vi "ErrorLog.vi"(7 "ErrorLogMode":T1=enum."Add", 8 "error in (no error)":errorcluster caption="エラー入力（エラーなし）", 10 "ModuleName":string="Manager") -> (0 "error out":errorcluster caption="エラー出力", 3 "path":path)   [LabVIEW 2021]
doc: "ErrorLogを保存します。\nInitモードで初期化時にログファイルを作成します。\nログファイルはユーザードキュメントフォルダ内の”ModuleName”のフォルダにErrorLog20210227.txtなどの名称で作成します。（20210527は作成年月日）\nAddモード時にエラー入力にエラーが入力されると上記ファイルに保存します。\n保存する項目は、日付_時刻（年月日_時分秒）、エラーCode、エラーソースです。\nエラーログファイルは、書き込み時に毎回、開く、閉じるの操作を行います。\n大量のエラーが連続して発生すると書き込み処理が追いつかなくなる恐れが有ります。"
uses:
  ErrorLogMode.ctl
  <vilib>/Utility/sysdir.llb/System Directory Type.ctl
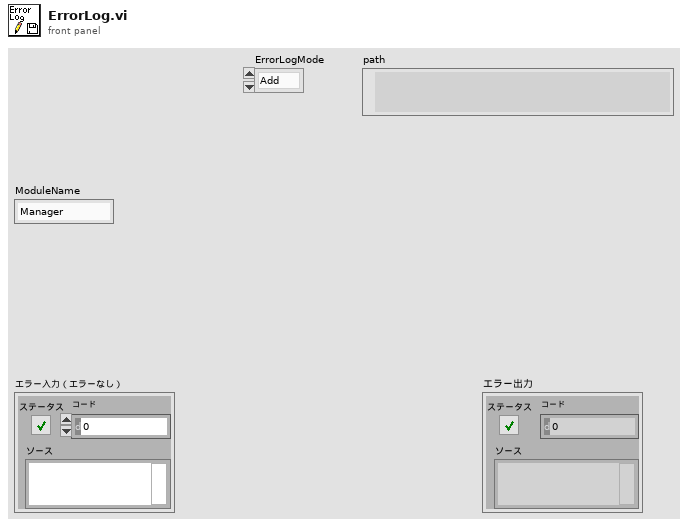
[diagram p1: front panel]
types:
  T1 = typedef "ErrorLogMode.ctl" = enum16{"Init", "Add"}
  T2 = enum16{"open", "replace", "create", "open or create", "replace or create", "replace or create with confirmation"}
  T3 = typedef "System Directory Type.ctl" = i32
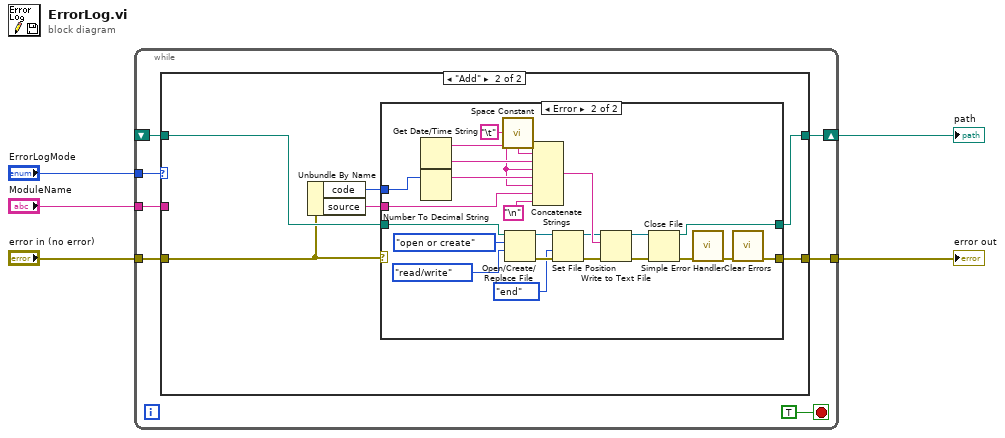
[diagram p0: block diagram]
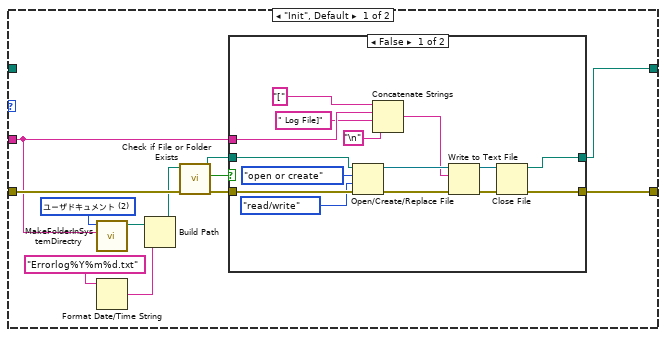
[diagram p2: hidden frame]
diagram:
  n1 = while {
    tunnel: "ErrorLogMode" -> [w11]
    tunnel: "error in (no error)" -> [w10]
    tunnel: [w9] -> w3
    shift-right: [w8] -> w1
    shift-left: _ -> [w7]
    tunnel: "ModuleName" -> [w6]
    stop <- TRUE stop-if-true
    n2 = case shown="\"Add\"" w11 {
      tunnel: w10 -> [w24 w42]
      tunnel: [w22 w47] -> w9
      tunnel: [w20 w46] -> w8
      tunnel: w7 -> [_ w43]
      tunnel: w6 -> [w13 _]
      frame "Init", Default {
        w15 = T3 2 items=["ユーザホーム"=0, "ユーザデスクトップ"=1, "ユーザドキュメント"=2, "ユーザアプリケーションデータ"=3, "ユーザ設定"=4, "ユーザ一時"=5, "パブリックドキュメント"=6, "パブリックアプリケーションデータ"=7, "パブリック環境設定"=8, "パブリックキャッシュ"=13, "システムコアライブラリ"=9, "システムインストールされたライブラリ"=10, "アプリケーションファイル"=11, "ブート容量ルート"=12] ("system directory type")
        n3 = call "MakeFolderInSystemDirectry.vi"("名前または相対パス"=w13, "system directory type"=w15) -> ("dup path"=w17:path)  [unwired: 8 in, 1 out]
        n4 = Format Date/Time String(time format string (%c)="Errorlog%Y%m%d.txt" ("名前または相対パス")) -> (date/time string=w18:string)  [unwired: 2 in]
        n5 = Build Path(base path=w17, name or relative path=w18) -> (appended path=w14:path)
        n6 = call <vilib>:"Check if File or Folder Exists.vi"("error in (no error)"=w24, "path"=w14) -> ("error out"=w21:errorcluster, "file or folder exists?"=w23:bool, "dup path"=w19:path)  [unwired: 7 in]
        n7 = case shown="False" w23 {
          tunnel: [w35 w41] -> w22
          tunnel: w21 -> [w39 w41]
          tunnel: [w32 w40] -> w20
          tunnel: w19 -> [w33 w40]
          tunnel: w13 -> [w27 _]
          frame False {
            n8 = Open/Create/Replace File(file path (use dialog)=w33, error in=w39, operation (0:open)=T2."open or create" ("操作（0:open）"), access (0:read/write)=enum16{"read/write", "read-only", "write-only"}."read/write" ("アクセス（0:read/write）")) -> (refnum out=w34:refnum<file>, error out=w38:errorcluster)  [unwired: 2 in, 1 out]
            n9 = Concatenate Strings("[" ("テキスト"), w27, " Log File]" ("文字列"), "\n") -> (w28:string)
            n10 = Write to Text File(file (use dialog)=w34, text=w28, error in=w38) -> (refnum out=w36:refnum<file>, error out=w37:errorcluster)  [unwired: 1 in, 1 out]
            n11 = Close File(refnum=w36, error in=w37) -> (path=w32:path, error out=w35:errorcluster)
          }
          frame True {
          }
        }
      }
      frame "Add" {
        n12 = Unbundle By Name(w42) -> ("code"=w45:i32, "source"=w44:string)
        n13 = case shown="Error" w42 {
          selector: w42 -> [w48 _]
          tunnel: [w48 w54] -> w47
          tunnel: [w49 w71] -> w46
          tunnel: w45 -> [_ w61]
          tunnel: w44 -> [_ w57]
          tunnel: w43 -> [w49 w56]
          frame No Error {
          }
          frame Error {
            w59 = "\t"
            n14 = Get Date/Time String() -> (date string=w63:string, time string=w64:string)  [unwired: 3 in]
            n15 = Number To Decimal String(number=w61) -> (decimal integer string=w60:string)  [unwired: 1 in]
            n16 = call <vilib>:"Space Constant.vi"() -> ("String"=w62:string)
            n17 = Open/Create/Replace File(file path (use dialog)=w56, operation (0:open)=T2."open or create" ("操作（0:open）"), access (0:read/write)=enum16{"read/write", "read-only", "write-only"}."read/write" ("アクセス（0:read/write）")) -> (refnum out=w68:refnum<file>, error out=w52:errorcluster)  [unwired: 3 in, 1 out]
            n18 = Concatenate Strings(w63, w62, w64, w59, w60, w59, w57, "\n") -> (w65:string)
            n19 = Set File Position(refnum=w68, from (0:start)=enum16{"start", "end", "current"}."end" ("基点（0:start）"), error in=w52) -> (refnum out=w53:refnum<file>, error out=w51:errorcluster)  [unwired: 1 in]
            n20 = Write to Text File(file (use dialog)=w53, text=w65, error in=w51) -> (refnum out=w69:refnum<file>, error out=w70:errorcluster)  [unwired: 1 in, 1 out]
            n21 = Close File(refnum=w69, error in=w70) -> (path=w71:path, error out=w72:errorcluster)
            n22 = call <vilib>:"Simple Error Handler.vi"("error in (no error)"=w72) -> ("error out"=w55:errorcluster)  [unwired: 4 in, 4 out]
            n23 = call <vilib>:"Clear Errors.vi"("error in (no error)"=w55) -> ("error out"=w54:errorcluster)  [unwired: 5 in, 1 out]
          }
        }
      }
    }
  }
  "error out" <- w3
  "path" <- w1
